vi "ChassisSpeeds_New.vi"(9 "vAngular":dbl, 10 "vY":dbl, 11 "vX":dbl) -> (3 "CHASSIS":T1 {"vOmega" format="%10.3f"; "vY" format="%10.3f"; "vX" format="%10.3f"})   [LabVIEW 2019, in "Trajectory_Library.lvlib"]
doc: "Constructs a ChassisSpeeds object.\n\nRepresents the speed of a robot chassis. Although this struct contains similar members compared to a Twist2d, they do NOT represent the same thing. Whereas a Twist2d represents a change in pose w.r.t to the robot frame of reference, this ChassisSpeeds struct represents a velocity w.r.t to the robot frame of\nreference.\n\nA strictly non-holonomic drivetrain, such as a differential drive, should never have a dy component because it can never move sideways. Holonomic drivetrains such as swerve and mecanum will often have all three components.\n\nParameters:\n - vx - Forward velocity. (Meters/Second)\n - vy - Sideways velocity. (Meters/Second)\n - omega - Angular velocity. (Radians/Second)\n\nReturns:\n - Chassis - CHASSIS_SPEEDS Data structure"
uses:
  Trajectory_Library.lvlib
  TypeDef/CHASSIS_SPEEDS.ctl
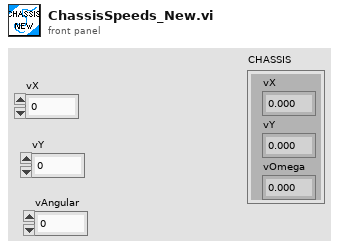
[diagram p1: front panel]
types:
  T1 = typedef "Trajectory_Library.lvlib/CHASSIS_SPEEDS.ctl" = cluster{"vX":dbl, "vY":dbl, "vOmega":dbl}
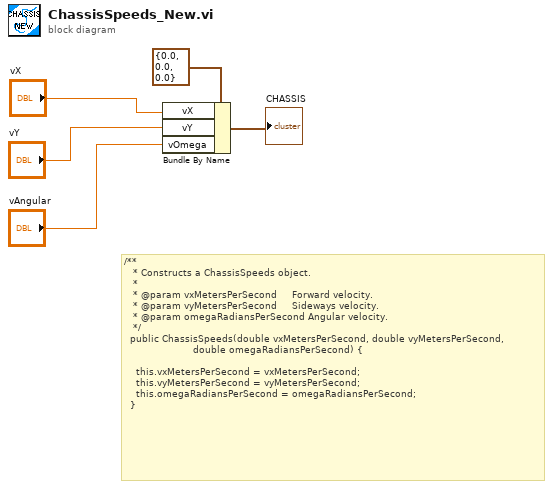
[diagram p0: block diagram]
diagram:
  # "/**\n   * Constructs a ChassisSpeeds object.\n   *\n   * @param vxMetersPerSecond     Forward velocity.\n   * @param vyMetersPerSecond     Sideways velocity.\n   * @param omegaRadiansPerSecond Angular velocity.\n   */\n  public ChassisSpeeds(double vxMetersPerSecond, double vyMetersPerSecond,\n                       double omegaRadiansPerSecond) {\n\n    this.vxMetersPerSecond = vxMetersPerSecond;\n    this.vyMetersPerSecond = vyMetersPerSecond;\n    this.omegaRadiansPerSecond = omegaRadiansPerSecond;\n  }"
  n1 = Bundle By Name(cluster=T1 {"vX"=0.0, "vY"=0.0, "vOmega"=0.0} ("CHASSIS"), "vX"="vX", "vY"="vY", "vOmega"="vAngular") -> (→"CHASSIS":T1)
